vi "Get Subroutine Info.vi"(11 "error in":errorcluster) -> (4 "data":T1, 15 "error out":errorcluster)   [LabVIEW 2021, in "Converter Reusables.lvlib"]
uses:
  Converter Reusables.lvlib
  TypeDefs/Error Information.ctl
  TypeDefs/Dictionary States.ctl
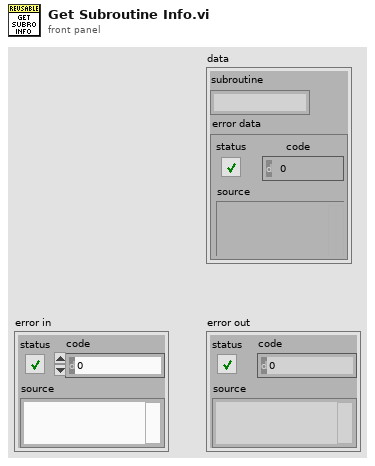
[diagram p1: front panel]
types:
  T1 = typedef "Converter Reusables.lvlib/Error Information.ctl" = cluster{"subroutine":string, "error data":errorcluster}
  T2 = typedef "Converter Reusables.lvlib/Dictionary States.ctl" = enum16{"Set", "Get", "Delete", "Delete All"}
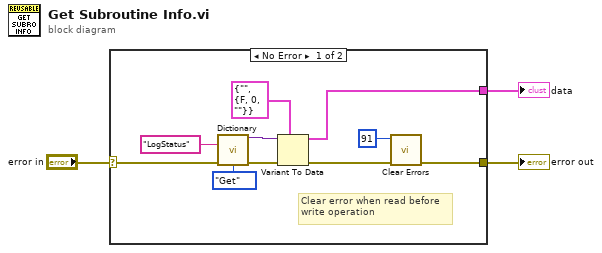
[diagram p0: block diagram]
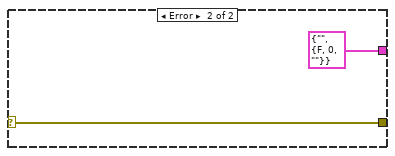
[diagram p2: hidden frame]
diagram:
  n1 = case shown="No Error" "error in" {
    selector: "error in" -> [w13 w14]
    tunnel: [w5 w14] -> w2
    tunnel: [w8 T1 {"subroutine"="", "error data"={"status"=FALSE, "code"=0, "source"=""}} ("ErrorInformation")] -> w1
    frame No Error {
      # "Clear error when read before\nwrite operation"
      n2 = call "Dictionary.vi"("key"="LogStatus" ("Key"), "error in"=w13, "dict states"=Dictionary_States."Get" ("Dict States")) -> ("variant out"=w11:variant, "error out"=w12:errorcluster)  [unwired: 11 in]
      n3 = Variant To Data(error in=w12, type=T1 {"subroutine"="", "error data"={"status"=FALSE, "code"=0, "source"=""}} ("ErrorInformation"), Variant=w11) -> (data=w8:T1, error out=w7:errorcluster)
      n4 = call <vilib>:"Clear Errors.vi"("error in (no error)"=w7, "specific error code to clear (0: all)"=91) -> ("error out"=w5:errorcluster)  [unwired: 4 in, 1 out]
    }
    frame Error {
    }
  }
  "error out" <- w2
  "data" <- w1
